vi "diff.vi"(9 "dt":dbl, 10 "x(n-1)":dbl, 11 "x(n)":dbl) -> (2 "x(n)":dbl, 3 "x_dot":dbl)   [LabVIEW 2017]
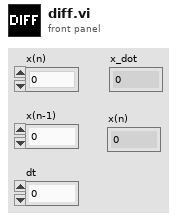
[diagram p1: front panel]
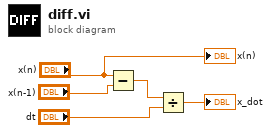
[diagram p0: block diagram]
diagram:
  n1 = Subtract(x="x(n)", y="x(n-1)") -> (x-y=w3:dbl)
  n2 = Divide(x=w3, y="dt") -> (x/y=→"x_dot":dbl)
  "x(n)" <- "x(n)"
